vi "UI Config.vi"(8 "error in (no error)":errorcluster, 10 "Actor Name":string, 11 "UI_Config in":refnum<class "UI_Config.lvclass">) -> (0 "error out":errorcluster, 3 "UI_Config out":refnum<class "UI_Config.lvclass">)   [LabVIEW 2021, in "UI_Config.lvlib" / "UI_Config.lvclass"]
uses:
  <userlib>/John_Lib/Interfaces/UI_Config/UI_Config.lvclass
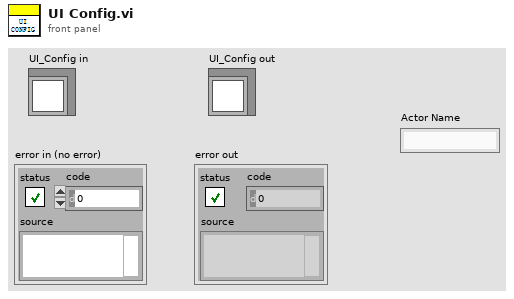
[diagram p1: front panel]
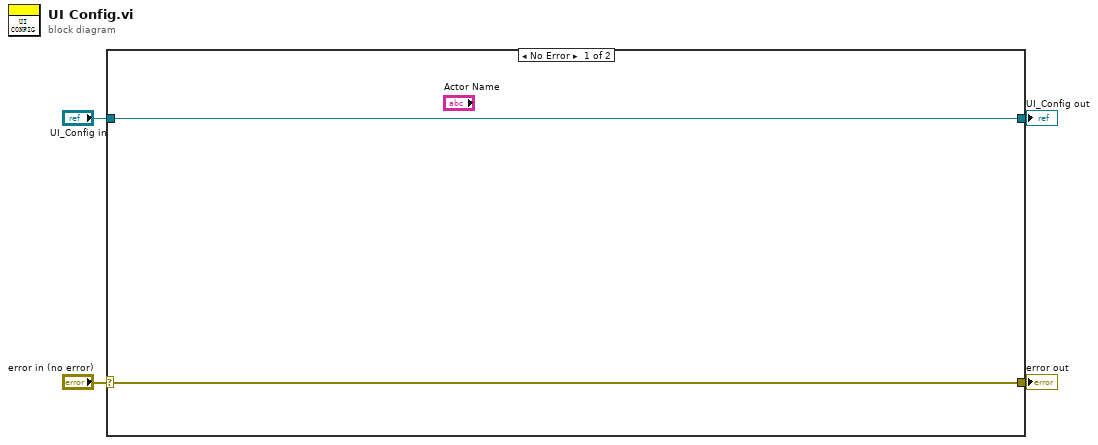
[diagram p0: block diagram]
diagram:
  n1 = case shown="No Error" "error in (no error)" {
    selector: "error in (no error)" -> [w5 w8]
    tunnel: [w5 w8] -> w3
    tunnel: [w6 w7] -> w1
    tunnel: "UI_Config in" -> [w6 w7]
    frame No Error {
    }
    frame Error {
    }
  }
  "error out" <- w3
  "UI_Config out" <- w1
